vi "Write Cluster.vi"(8 "error in (no error)":errorcluster, 10 "Cluster":T1={"VideoMode"=0, "gain"=6818, "gamma"=0.43, "Contrast"=37.81818181818181, "Exposure"=32, "Saturation"=6818} {"Saturation" max=7764 scale=0.0..7764.0; "Exposure" scale=1.0..2048.0; "Contrast" min=0.0 max=78.0 scale=0.0..78.0 scale format="%.2f"; "gamma" min=0.43 max=5 scale=0.43..5.0; "gain" min=1000 max=7000 scale=1000.0..7000.0; "VideoMode" items=["640x480 RGB24 30FPS", "1024x768 RGB24 18FPS", "1920x1080 RGB24  10FPS", "2048x1536 RGB24 3FPS"]}, 11 "CCD in":refnum<class "CCD.lvclass">) -> (0 "error out":errorcluster, 3 "CCD out":refnum<class "CCD.lvclass">)   [LabVIEW 2016, in "CCD.lvlib" / "CCD.lvclass"]
uses:
  <userlib>/Common Components/Hardware/CCD/CCD/CCD.lvclass
  <userlib>/Common Components/Hardware/CCD/CCD/camer data.ctl
  <userlib>/Common Components/Hardware/CCD/CCD/CCD.lvclass/CCD.ctl
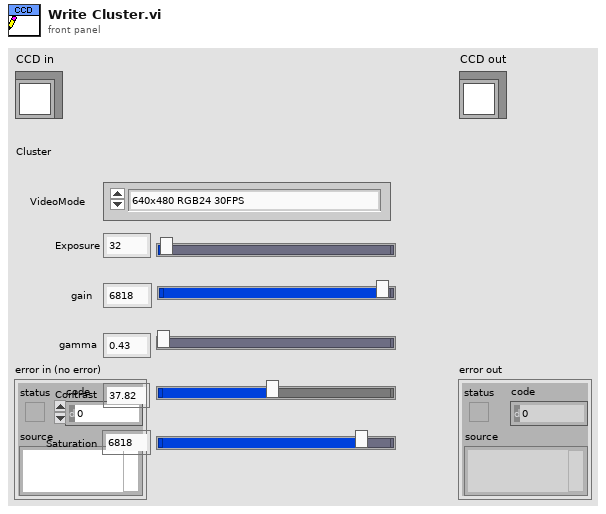
[diagram p1: front panel]
types:
  T1 = typedef "CCD.lvlib/CCD.lvclass/camer data.ctl" = cluster{"VideoMode":u16, "gain":u32, "gamma":sgl, "Contrast":dbl, "Exposure":u32, "Saturation":u32}
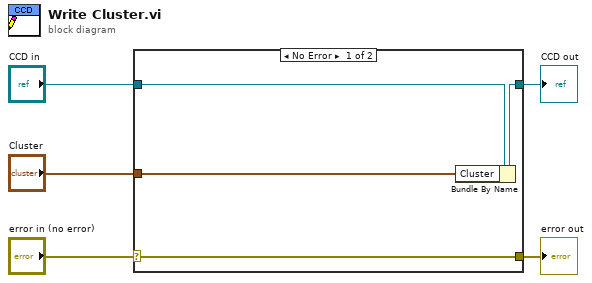
[diagram p0: block diagram]
diagram:
  n1 = case shown="No Error" "error in (no error)" {
    selector: "error in (no error)" -> [w9 w10]
    tunnel: [w9 w10] -> w4
    tunnel: [w7 w11] -> w2
    tunnel: "CCD in" -> [w8 w11]
    tunnel: "Cluster" -> [w6 _]
    frame No Error {
      n2 = Bundle By Name(cluster=w8, "Cluster"=w6) -> (w7:refnum<class "CCD.lvclass">)
    }
    frame Error {
    }
  }
  "error out" <- w4
  "CCD out" <- w2
